vi "S2C_SetBreakOnFail.vi"(8 "Error In":errorcluster, 11 "MenuRef":refnum<k9>) -> (0 "Error Out":errorcluster)   [LabVIEW 2015]
doc: "Toggles the \"Local File\" runtime menu item."
uses:
  Globals/S2C_Globals.vi
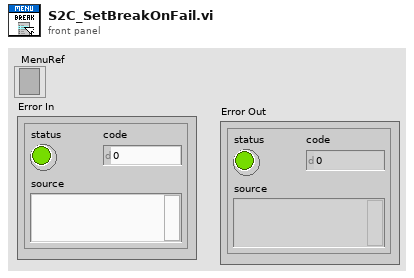
[diagram p1: front panel]
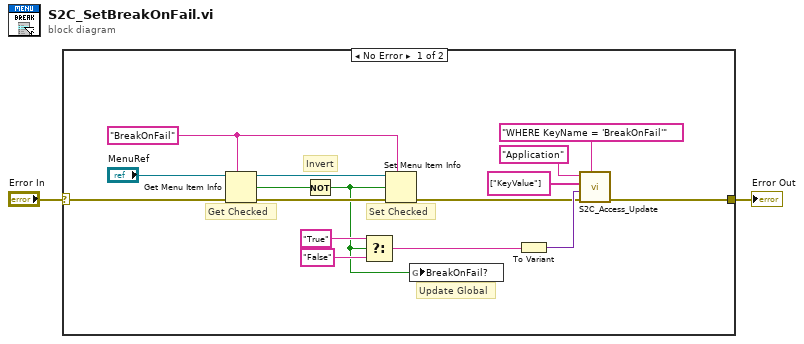
[diagram p0: block diagram]
diagram:
  n1 = case shown="No Error" "Error In" {
    selector: "Error In" -> [w7 w19]
    tunnel: [w6 w19] -> w1
    frame No Error {
      w4 = "BreakOnFail" ("item tag")
      # "Update Global"
      # "Invert"
      # "Set Checked"
      # "Get Checked"
      n2 = Get Menu Item Info(7:w4, 8:w7, 11:"MenuRef") -> (0:w18:errorcluster, 3:w17:refnum<k9>, 4:w16:bool)  [unwired: 4 out]
      n3 = Not(x=w16) -> (.not. x?=w3:bool)
      n4 = Select(t="True", s=w3, f="False") -> (s? t:f=w8:string)
      n5 = Set Menu Item Info(6:w3, 7:w4, 8:w18, 11:w17) -> (0:w9:errorcluster)  [unwired: 3 in, 1 out]
      n6 = global write "S2C_Globals.vi" "BreakOnFail?"(w3) -> ()
      n7 = To Variant(anything=w8) -> (Variant=w11:variant)
      n8 = call "S2C_Access_Update.vi"("Condition"="WHERE KeyName = 'BreakOnFail'", "Error In"=w9, "Data"=w11, "Columns"=string[] ["KeyValue"], "Table"="Application") -> ("Error Out"=w6:errorcluster)  [unwired: 6 in]
    }
    frame Error {
    }
  }
  "Error Out" <- w1
